vi "Send Response.vi"(8 "error in (no error)":errorcluster, 10 "command in":T1, 11 "Dispatcher in":refnum<class "Dispatcher.lvclass">) -> (0 "error out":errorcluster, 2 "command out":T1, 3 "Dispatcher out":refnum<class "Dispatcher.lvclass">)   [LabVIEW 2017, in "DSF Core.lvlib" / "Dispatcher.lvclass"]
uses:
  Dispatcher.lvclass
  Interfaces/Dispatcher/Dispatcher Interface.lvclass
  Interfaces/Dispatcher/Response.ctl
  Interfaces/Dispatcher/Response Data.ctl
  Interfaces/Dispatcher/Parameters.ctl
  C:/Git/DSF/Data Sharing Framework/Source/Core/Engine/Classes/Interfaces/Interface/Interface.lvclass
  Interfaces/Dispatcher/Command.ctl
  Interfaces/Dispatcher/Command Data.ctl
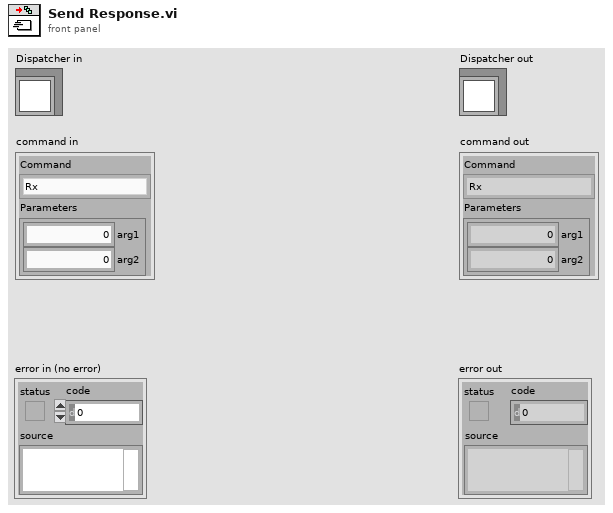
[diagram p1: front panel]
types:
  T1 = typedef "DSF Core.lvlib/Dispatcher Interface.lvclass/Command Data.ctl" = cluster{"Command":T2, "Parameters":T3}
  T2 = typedef "DSF Core.lvlib/Dispatcher Interface.lvclass/Command.ctl" = enum8{"Rx", "Tx", "Shutdown"}
  T3 = typedef "DSF Core.lvlib/Dispatcher Interface.lvclass/Parameters.ctl" = cluster{"arg1":u64, "arg2":u64}
  T4 = typedef "DSF Core.lvlib/Dispatcher Interface.lvclass/Response Data.ctl" = cluster{"Response":T5, "Parameters":T3}
  T5 = typedef "DSF Core.lvlib/Dispatcher Interface.lvclass/Response.ctl" = enum8{"General Ack", "Error", "Shutting Down"}
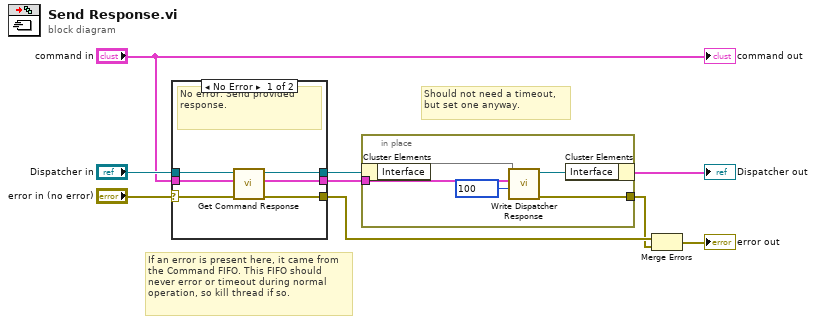
[diagram p0: block diagram]
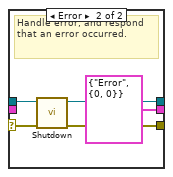
[diagram p2: hidden frame]
diagram:
  # "If an error is present here, it came from the Command FIFO. This FIFO should never error or timeout during normal operation, so kill thread if so."
  # "Should not need a timeout, but set one anyway."
  n1 = case shown="No Error" "error in (no error)" {
    selector: "error in (no error)" -> [w10 w18]
    tunnel: "Dispatcher in" -> [w15 w19]
    tunnel: [w14 w16] -> w6
    tunnel: [w13 w17] -> w3
    tunnel: [w12 T4 {"Response"=enum."Error", "Parameters"={"arg1"=0, "arg2"=0}} ("Dispatcher Response")] -> w4
    tunnel: "command in" -> [w11 _]
    frame No Error {
      # "No error. Send provided response."
      n2 = call "Get Command Response.vi"("error in (no error)"=w10, "command"=w11, "Dispatcher Interface in"=w15) -> ("error out"=w13:errorcluster, "response"=w12:T4, "Dispatcher Interface out"=w14:refnum<class "Dispatcher Interface.lvclass">)  [unwired: 6 in]
    }
    frame Error {
      # "Handle error, and respond that an error occurred."
      n3 = call "Shutdown.vi"("error in (no error)"=w18, "Dispatcher in"=w19) -> ("error out"=w17:errorcluster, "Dispatcher out"=w16:refnum<class "Dispatcher.lvclass">)  [unwired: 8 in]
    }
  }
  n4 = in-place {
    in-place-border: [w24] -> w2
    in-place-border: w4 -> [w21]
    n5 = in-place-cluster #1(w6) -> ("Interface"=w23)
    n6 = call "Write Dispatcher Response.vi"("timeout in ms (0)"=100, "response"=w21, "Dispatcher Interface in"=w23) -> ("error out"=w24:errorcluster, "Dispatcher Interface out"=w22:refnum<class "Dispatcher Interface.lvclass">)  [unwired: 6 in, 1 out]
    n7 = in-place-cluster #1("Interface"=w22) -> (→"Dispatcher out":cluster{})
  }
  n8 = Merge Errors(w3, w2) -> (→"error out":errorcluster)
  "command out" <- "command in"
